vi "Update Listbox Symbols.vi"(8 "error in (no error)":errorcluster, 9 "Operation":T1(ring), 10 "Indices to change":i32[](array[numeric]), 11 "ListBox in":refnum<vi>) -> (0 "error out":errorcluster, 3 "ListBox out":refnum<vi>)   [LabVIEW 2023, in "SwitchExecController.lvlib"]
uses:
  SwitchExecController.lvlib
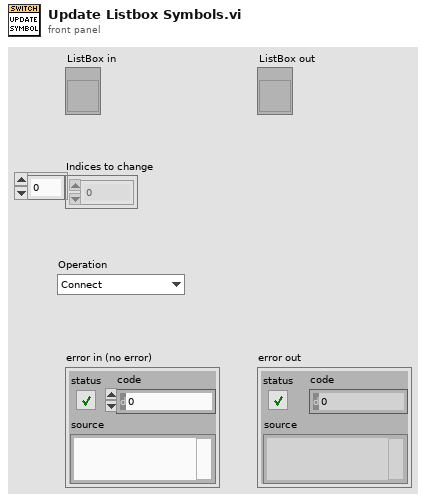
[diagram p1: front panel]
types:
  T1 = enum16{"Connect", "Disconnect", "Disconnect All"}
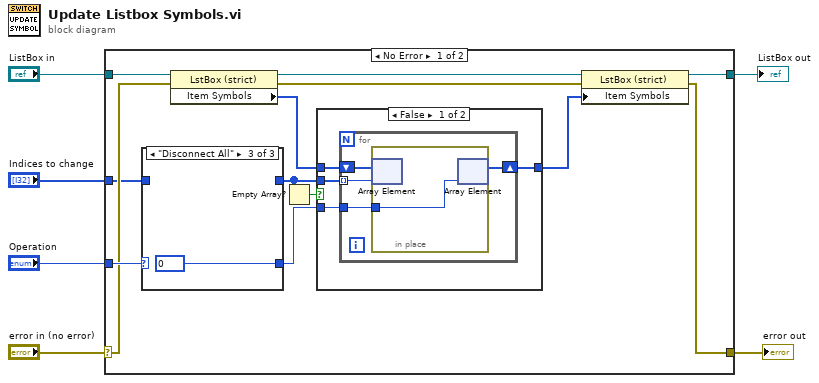
[diagram p0: block diagram]
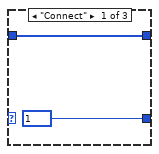
[diagram p2: hidden frame]
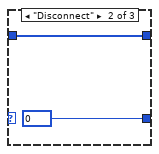
[diagram p3: hidden frame]
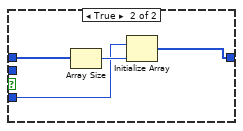
[diagram p4: hidden frame]
diagram:
  n1 = case shown="No Error" "error in (no error)" {
    selector: "error in (no error)" -> [w11 w39]
    tunnel: "ListBox in" -> [w19 w38]
    tunnel: "Operation" -> [w14 _]
    tunnel: "Indices to change" -> [w7 _]
    tunnel: [w10 w39] -> w3
    tunnel: [w9 w38] -> w2
    frame No Error {
      n2 = case shown="\"Disconnect All\"" w14 {
        tunnel: [1 0 0] -> w13
        tunnel: [w20 w22 _] -> w8
        tunnel: w7 -> [w20 w22 _]
        frame "Connect" {
        }
        frame "Disconnect" {
        }
        frame "Disconnect All" {
        }
      }
      n3 = property on="Property Node" class="LstBox (strict)"(reference=w19, error in=w11) -> (reference out=w15:refnum<vi>, error out=w16:errorcluster, "Item Symbols"=w17:i32[])
      n4 = Empty Array?(array=w8) -> (empty?=w12:bool)
      n5 = case shown="False" w12 {
        tunnel: [w28 w34] -> w18
        tunnel: w17 -> [w27 w37]
        tunnel: w13 -> [w26 w35]
        tunnel: w8 -> [w25 _]
        frame False {
          n6 = for {
            shift-right: [w32] -> w28
            shift-left: w27 -> [w31]
            tunnel: w25 -> [w30] mode=indexing
            tunnel: w26 -> [w29]
            n7 = in-place {
              in-place-border: w29 -> [w33]
              n8 = in-place-array #1(w31, w30) -> ()  [unwired: 1 out]
              n9 = in-place-array #1(w33) -> (w32:i32[])  [unwired: 1 out]
            }
          }
        }
        frame True {
          n10 = Array Size(array=w37) -> (size(s)=w36:i32)
          n11 = Initialize Array(w35, w36) -> (w34:i32[])
        }
      }
      n12 = property on="Property Node" class="LstBox (strict)"(reference=w15, error in=w16, "Item Symbols"=w18) -> (reference out=w9:refnum<vi>, error out=w10:errorcluster)
    }
    frame Error {
    }
  }
  "error out" <- w3
  "ListBox out" <- w2
